vi "_Postprocess HTML file.vi"(0 "HTML File Path":path, 7 "VI Info":T1={"_vi_name_"="", "_vi_description_text_"="", "_vi_controls_and_indicators_descriptions_"="", "_name_of_owning_library_"="", "_owning_library_html_"="", "_Packages_"="Base Package", "_Platforms_"="Windows", "_details_text_"="Put details here", "_example_screenshot_"="", "_example_vi_"="", "_path_to_example_file_"=path "", "IsDetailsON?"=FALSE, "IsOwningLibraryON?"=FALSE, "IsExamplesON?"=FALSE, "IsTableON?"=FALSE, "IsScrollableON?"=FALSE, "IsDetailedHelpLinkON?"=FALSE, "Table Objects array"=[], "Table Descriptions array"=[], "Table Links array"=[], "Start path location"=enum."VI folder"}, 11 "error in":errorcluster) -> (4 "HTML File Path out":path, 15 "error out":errorcluster)   [LabVIEW 2012]
uses:
  _Controls and TypeDefs/InfoFromOldHTML_cluster.ctl
  _Controls and TypeDefs/StartPathLocation_enum.ctl
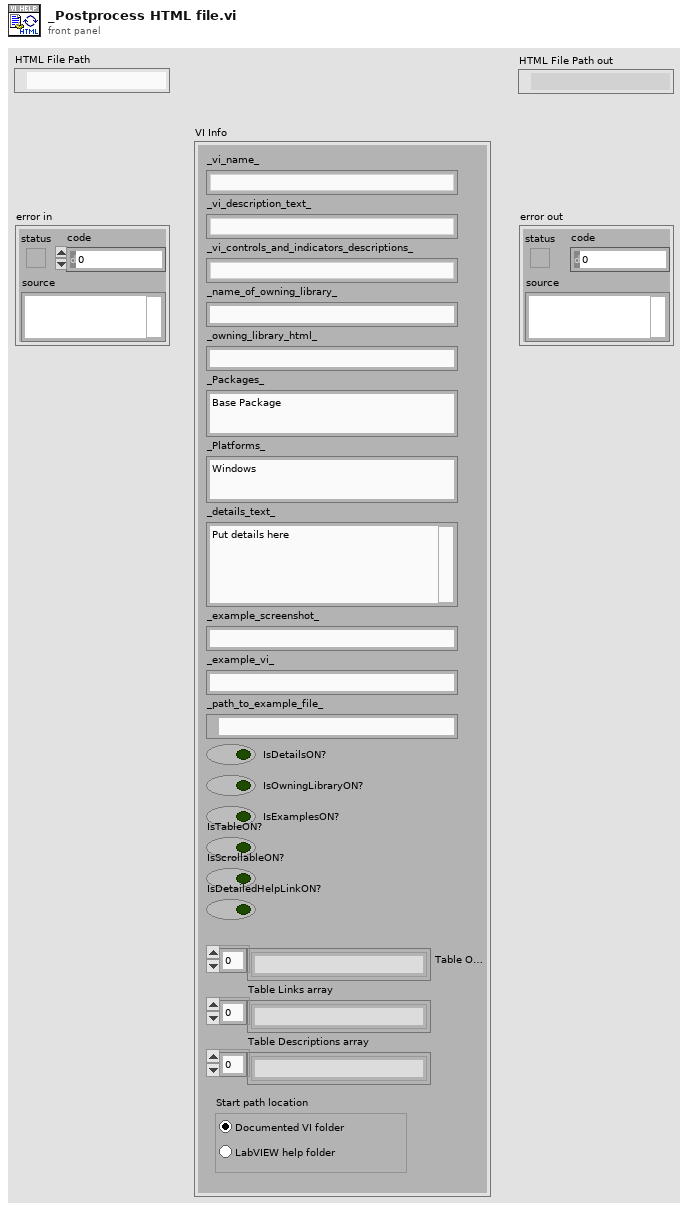
[diagram p1: front panel]
types:
  T1 = typedef "InfoFromOldHTML_cluster.ctl" = cluster{"_vi_name_":string, "_vi_description_text_":string, "_vi_controls_and_indicators_descriptions_":string, "_name_of_owning_library_":string, "_owning_library_html_":string, "_Packages_":string, "_Platforms_":string, "_details_text_":string, "_example_screenshot_":string, "_example_vi_":string, "_path_to_example_file_":path, "IsDetailsON?":bool, "IsOwningLibraryON?":bool, "IsExamplesON?":bool, "IsTableON?":bool, "IsScrollableON?":bool, "IsDetailedHelpLinkON?":bool, "Table Objects array":string[], "Table Descriptions array":string[], "Table Links array":string[], "Start path location":T2}
  T2 = typedef "StartPathLocation_enum.ctl" = enum32{"VI folder", "Help folder"}
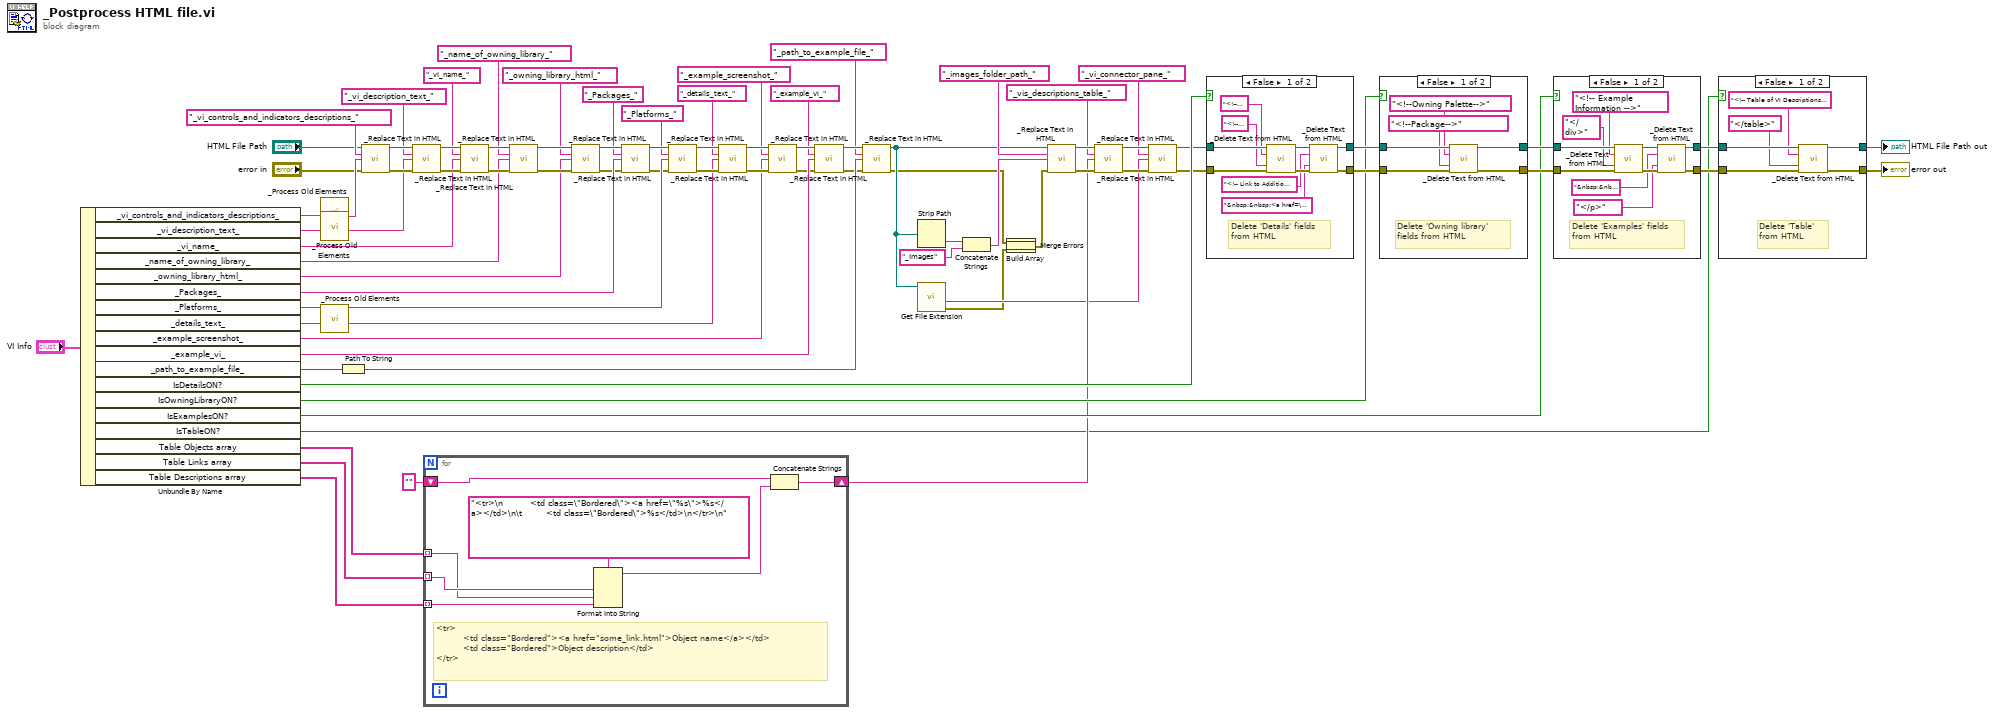
[diagram p0: block diagram]
diagram:
  n1 = Unbundle By Name("VI Info") -> ("_vi_controls_and_indicators_descriptions_"=w39:string, "_vi_description_text_"=w37:string, "_vi_name_"=w78:string, "_name_of_owning_library_"=w74:string, "_owning_library_html_"=w20:string, "_Packages_"=w72:string, "_Platforms_"=w71:string, "_details_text_"=w19:string, "_example_screenshot_"=w21:string, "_example_vi_"=w70:string, "_path_to_example_file_"=w73:path, "IsDetailsON?"=w46:bool, "IsOwningLibraryON?"=w41:bool, "IsExamplesON?"=w40:bool, "IsTableON?"=w2:bool, "Table Objects array"=w26:string[], "Table Links array"=w25:string[], "Table Descriptions array"=w24:string[])
  n2 = call "_Process Old Elements.vi"("Input Text"=w39) -> ("Processed Text"=w38:string)  [unwired: 8 in, 1 out]
  n3 = call "_Process Old Elements.vi"("Input Text"=w37) -> ("Processed Text"=w36:string)  [unwired: 8 in, 1 out]
  n4 = call "_Process Old Elements.vi"("Input Text"=w19) -> ("Processed Text"=w18:string)  [unwired: 8 in, 1 out]
  n5 = Path To String(path=w73) -> (string=w69:string)
  n6 = call "_Replace Text in HTML.vi"("HTML File Path"="HTML File Path", "search string"="_vi_controls_and_indicators_descriptions_" ("replace string (\"\")"), "replace string (\"\")"=w38, "error in"="error in") -> ("HTML File Path out"=w80:path, "error out"=w81:errorcluster)  [unwired: 10 in]
  n7 = call "_Replace Text in HTML.vi"("HTML File Path"=w80, "search string"="_vi_description_text_" ("replace string (\"\")"), "replace string (\"\")"=w36, "error in"=w81) -> ("HTML File Path out"=w84:path, "error out"=w83:errorcluster)  [unwired: 10 in]
  n8 = for {
    tunnel: w26 -> [w90] mode=indexing
    tunnel: w25 -> [w91] mode=indexing
    tunnel: w24 -> [w89] mode=indexing
    shift-right: [w86] -> w22
    shift-left: "" -> [w88]
    # "<tr>\n         <td class=\"Bordered\"><a href=\"some_link.html\">Object name</a></td>\n\t        <td class=\"Bordered\">Object description</td>\n</tr>"
    n9 = Format Into String(format string="<tr>\n         <td class=\"Bordered\"><a href=\"%s\">%s</a></td>\n\t        <td class=\"Bordered\">%s</td>\n</tr>\n", w91, w90, w89) -> (resulting string=w87:string)  [unwired: 2 in, 1 out]
    n10 = Concatenate Strings(w88, w87) -> (w86:string)
  }
  n11 = call "_Replace Text in HTML.vi"("HTML File Path"=w84, "search string"="_vi_name_" ("replace string (\"\")"), "replace string (\"\")"=w78, "error in"=w83) -> ("HTML File Path out"=w76:path, "error out"=w75:errorcluster)  [unwired: 10 in]
  n12 = call "_Replace Text in HTML.vi"("HTML File Path"=w76, "search string"="_name_of_owning_library_" ("replace string (\"\")"), "replace string (\"\")"=w74, "error in"=w75) -> ("HTML File Path out"=w65:path, "error out"=w67:errorcluster)  [unwired: 10 in]
  n13 = call "_Replace Text in HTML.vi"("HTML File Path"=w65, "search string"="_owning_library_html_" ("replace string (\"\")"), "replace string (\"\")"=w20, "error in"=w67) -> ("HTML File Path out"=w64:path, "error out"=w66:errorcluster)  [unwired: 10 in]
  n14 = call "_Replace Text in HTML.vi"("HTML File Path"=w64, "search string"="_Packages_" ("replace string (\"\")"), "replace string (\"\")"=w72, "error in"=w66) -> ("HTML File Path out"=w63:path, "error out"=w62:errorcluster)  [unwired: 10 in]
  n15 = call "_Replace Text in HTML.vi"("HTML File Path"=w63, "search string"="_Platforms_" ("replace string (\"\")"), "replace string (\"\")"=w71, "error in"=w62) -> ("HTML File Path out"=w57:path, "error out"=w61:errorcluster)  [unwired: 10 in]
  n16 = call "_Replace Text in HTML.vi"("HTML File Path"=w57, "search string"="_details_text_" ("replace string (\"\")"), "replace string (\"\")"=w18, "error in"=w61) -> ("HTML File Path out"=w56:path, "error out"=w60:errorcluster)  [unwired: 10 in]
  n17 = call "_Replace Text in HTML.vi"("HTML File Path"=w56, "search string"="_example_screenshot_" ("replace string (\"\")"), "replace string (\"\")"=w21, "error in"=w60) -> ("HTML File Path out"=w55:path, "error out"=w59:errorcluster)  [unwired: 10 in]
  n18 = call "_Replace Text in HTML.vi"("HTML File Path"=w55, "search string"="_example_vi_" ("replace string (\"\")"), "replace string (\"\")"=w70, "error in"=w59) -> ("HTML File Path out"=w48:path, "error out"=w58:errorcluster)  [unwired: 10 in]
  n19 = call "_Replace Text in HTML.vi"("HTML File Path"=w48, "search string"="_path_to_example_file_" ("replace string (\"\")"), "replace string (\"\")"=w69, "error in"=w58) -> ("HTML File Path out"=w16:path, "error out"=w8:errorcluster)  [unwired: 10 in]
  n20 = Strip Path(path=w16) -> (name=w17:string)  [unwired: 1 out]
  n21 = call <vilib>:"Get File Extension.vi"("file"=w16) -> ("error out"=w9:errorcluster, "filename without extension"=w10:string)  [unwired: 7 in, 2 out]
  n22 = Concatenate Strings(w17, "_Images" ("string")) -> (w33:string)
  n23 = Build Array(w8, w9) -> (w1:errorcluster[])
  n24 = Merge Errors(w1) -> (w7:errorcluster)
  n25 = call "_Replace Text in HTML.vi"("HTML File Path"=w16, "search string"="_images_folder_path_" ("replace string (\"\")"), "replace string (\"\")"=w33, "error in"=w7) -> ("HTML File Path out"=w28:path, "error out"=w29:errorcluster)  [unwired: 10 in]
  n26 = call "_Replace Text in HTML.vi"("HTML File Path"=w28, "search string"="_vis_descriptions_table_", "replace string (\"\")"=w22, "error in"=w29) -> ("HTML File Path out"=w14:path, "error out"=w15:errorcluster)  [unwired: 10 in]
  n27 = call "_Replace Text in HTML.vi"("HTML File Path"=w14, "search string"="_vi_connector_pane_", "replace string (\"\")"=w10, "error in"=w15) -> ("HTML File Path out"=w12:path, "error out"=w13:errorcluster)  [unwired: 10 in]
  n28 = case shown="False" w46 {
    tunnel: w12 -> [w101 w103]
    tunnel: [w98 w103] -> w44
    tunnel: [w97 w102] -> w45
    tunnel: w13 -> [w96 w102]
    frame False {
      # "Delete 'Details' fields\nfrom HTML"
      n29 = call "_Delete Text from HTML.vi"("HTML File Path"=w101, "Text Before Delete"="<!-- Additional VI/Function Information -->", "Text After Delete"="<!-- Example Information -->", "error in"=w96) -> ("HTML File Path out"=w99:path, "error out"=w100:errorcluster)  [unwired: 10 in]
      n30 = call "_Delete Text from HTML.vi"("HTML File Path"=w99, "Text Before Delete"="<!-- Link to Additional VI/Function Information and Examples  -->\n\n<p class=\"Body\">", "Text After Delete"="&nbsp;&nbsp;<a href=\"#examples\">Example</a></p>", "error in"=w100) -> ("HTML File Path out"=w98:path, "error out"=w97:errorcluster)  [unwired: 10 in]
    }
    frame True {
    }
  }
  n31 = case shown="False" w41 {
    tunnel: w44 -> [w109 w111]
    tunnel: [w105 w111] -> w42
    tunnel: [w104 w110] -> w43
    tunnel: w45 -> [w108 w110]
    frame False {
      # "Delete 'Owning library' \nfields from HTML"
      n32 = call "_Delete Text from HTML.vi"("HTML File Path"=w109, "Text Before Delete"="<!--Owning Palette-->", "Text After Delete"="<!--Package-->", "error in"=w108) -> ("HTML File Path out"=w105:path, "error out"=w104:errorcluster)  [unwired: 10 in]
    }
    frame True {
    }
  }
  n33 = case shown="False" w40 {
    tunnel: w42 -> [w121 w123]
    tunnel: [w118 w123] -> w6
    tunnel: [w117 w122] -> w5
    tunnel: w43 -> [w116 w122]
    frame False {
      # "Delete 'Examples' fields\nfrom HTML"
      n34 = call "_Delete Text from HTML.vi"("HTML File Path"=w121, "Text Before Delete"="<!-- Example Information -->", "Text After Delete"="</div>", "error in"=w116) -> ("HTML File Path out"=w119:path, "error out"=w120:errorcluster)  [unwired: 10 in]
      n35 = call "_Delete Text from HTML.vi"("HTML File Path"=w119, "Text Before Delete"="&nbsp;&nbsp;", "Text After Delete"="</p>", "error in"=w120) -> ("HTML File Path out"=w118:path, "error out"=w117:errorcluster)  [unwired: 10 in]
    }
    frame True {
    }
  }
  n36 = case shown="False" w2 {
    tunnel: w6 -> [w129 w131]
    tunnel: [w125 w131] -> w4
    tunnel: [w124 w130] -> w3
    tunnel: w5 -> [w128 w130]
    frame False {
      # "Delete 'Table' \nfrom HTML"
      n37 = call "_Delete Text from HTML.vi"("HTML File Path"=w129, "Text Before Delete"="<!-- Table of VI Descriptions -->", "Text After Delete"="</table>", "error in"=w128) -> ("HTML File Path out"=w125:path, "error out"=w124:errorcluster)  [unwired: 10 in]
    }
    frame True {
    }
  }
  "error out" <- w3
  "HTML File Path out" <- w4
